vi "Module_IOWrite.vi"(7 "IOWrite_Cmd":T3, 8 "error in (no error)":errorcluster caption="エラー入力", 9 "IOName-LineName":cluster{"IOName":string, "DAQmxChannel":tag}[](array[cluster])=[{"IOName"="BPS_ON", "DAQmxChannel"="PXI1Slot4/port4/line7"}], 10 "ON/OFF":bool, 11 "IOName":string) -> (0 "error out":errorcluster caption="エラー出力", 2 "Check":bool, 3 "IO_State":T1(array[cluster]))   [LabVIEW 2018]
doc: "Module_IOWrite.vi\nIO信号のON/OFF切替を行う。\n\n◆IOWrite_Cmd=Init\n　IO信号制御用DOの初期化処理を行う。\n　また、入力のIO名とLine名の対応を保持する。\n　・Input：IOName-LineName\n\n◆IOWrite_Cmd=Set\n　入力のIONameの信号のON/OFFを切替。\n　・Input：IOName\n　　　　　 ON/OFF\n\n◆IOWrite_Cmd=ALL_OFF\n　全てのIONameの信号をOFFにする。\n\n◆IOWrite_Cmd=Check\n　現在のIO信号の状態を読み出す\n　・Output：IO_State\n\n◆IOWrite_Cmd=Close\n　IO信号信号制御用DOのクローズ処理を行う。"
uses:
  Ctl_IOWriteCommand.ctl
  <vilib>/DAQmx/read.llb/DAQmx Read (Digital 1D Bool NChan 1Samp 1Line).vi
  <vilib>/DAQmx/write.llb/DAQmx Write (Digital 1D Bool NChan 1Samp 1Line).vi
  <vilib>/DAQmx/create/channels.llb/DAQmx Create Channel (DO-Digital Output).vi
  <vilib>/DAQmx/miscellaneous.llb/DAQmx Fill In Error Info.vi
panel:
  in  "IOState":T2={"IOName"="AUTO", "DAQmxChannel"="PXI1Slot4/port0/line0", "ON/OFF"=FALSE}
  # "Output"
  # "Local"
  # "Input"
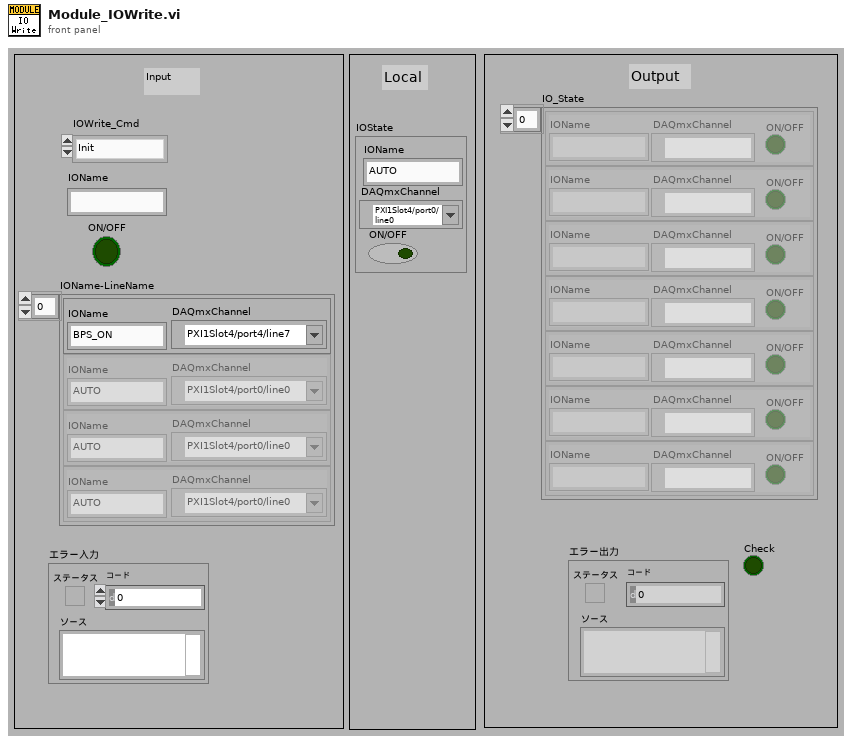
[diagram p1: front panel]
types:
  T1 = cluster{"IOName":string, "DAQmxChannel":tag, "ON/OFF":bool}[]
  T2 = cluster{"IOName":string, "DAQmxChannel":tag, "ON/OFF":bool}
  T3 = typedef "Ctl_IOWriteCommand.ctl" = enum16{"Init", "Set", "ALL_OFF", "Check", "Close"}
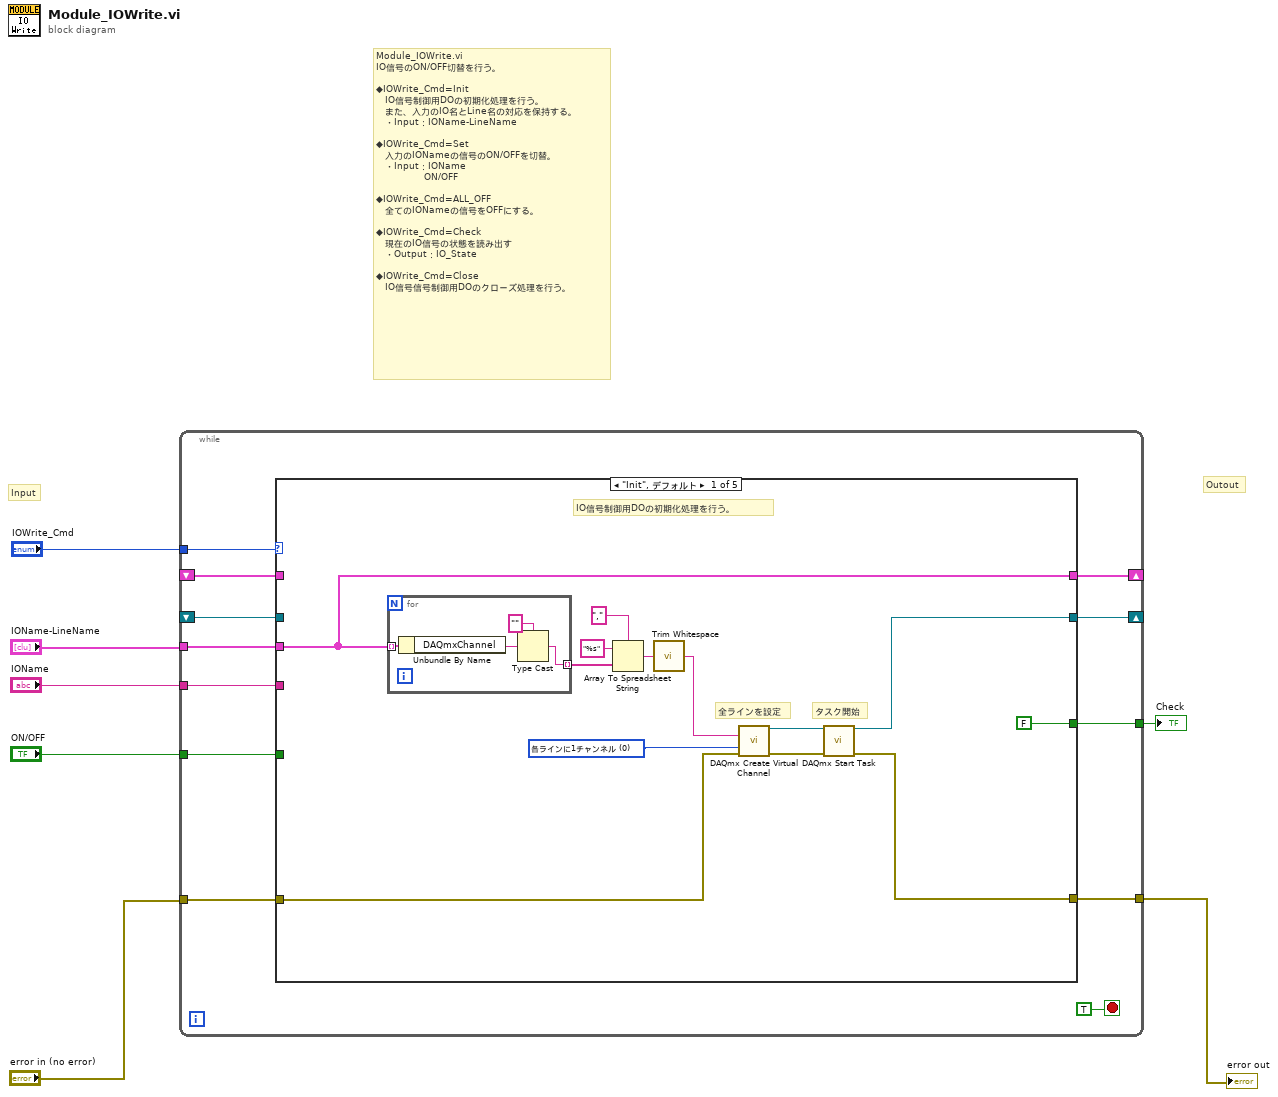
[diagram p0: block diagram]
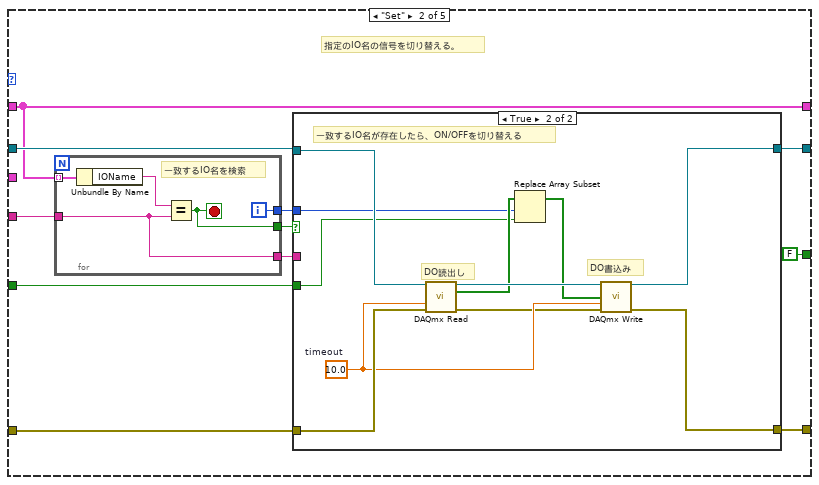
[diagram p2: hidden frame]
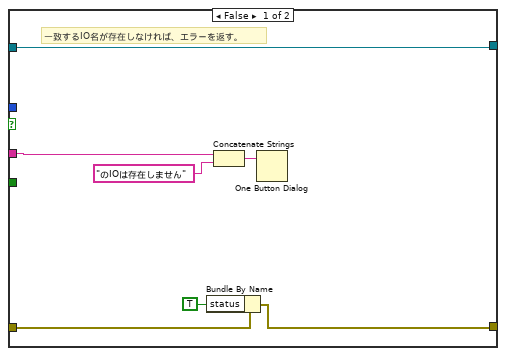
[diagram p3: hidden frame]
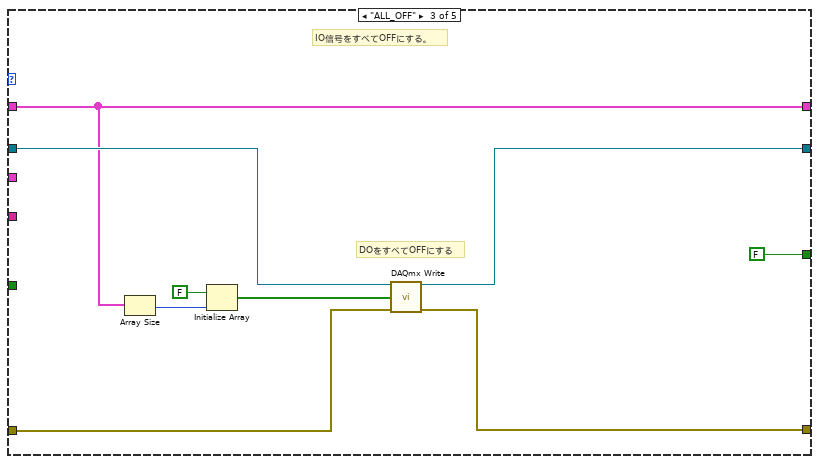
[diagram p4: hidden frame]
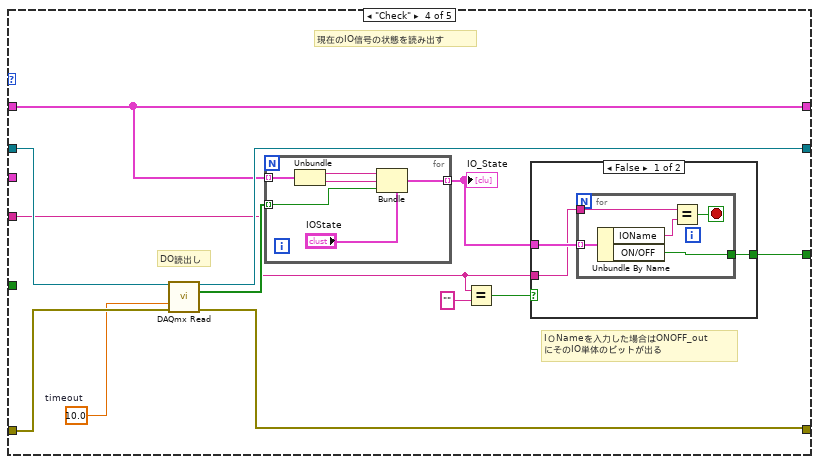
[diagram p5: hidden frame]
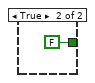
[diagram p6: hidden frame]
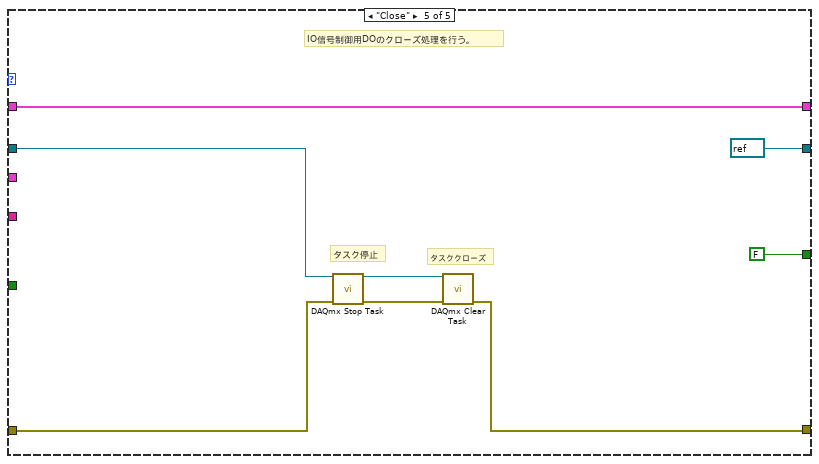
[diagram p7: hidden frame]
diagram:
  # "Module_IOWrite.vi\nIO信号のON/OFF切替を行う。\n\n◆IOWrite_Cmd=Init\n　IO信号制御用DOの初期化処理を行う。\n　また、入力のIO名とLine名の対応を保持する。\n　・Input：IOName-LineName\n\n◆IOWrite_Cmd=Set\n　入力のIONameの信号のON/OFFを切替。\n　・Input：IOName\n　　　　　 ON/OFF\n\n◆IOWrite_Cmd=ALL_OFF\n　全てのIONameの信号をOFFにする。\n\n◆IOWrite_Cmd=Check\n　現在のIO信号の状態を読み出す\n　・Output：IO_State\n\n◆IOWrite_Cmd=Close\n　IO信号信号制御用DOのクローズ処理を行う。"
  # "Outout"
  # "Input"
  n1 = while {
    tunnel: "error in (no error)" -> [w19]
    tunnel: "IOWrite_Cmd" -> [w18]
    shift-right: [w16] -> _
    shift-left: _ -> [w15]
    tunnel: [w8] -> w1
    tunnel: "ON/OFF" -> [w14]
    tunnel: "IOName-LineName" -> [w13]
    tunnel: "IOName" -> [w12]
    shift-right: [w11] -> _
    shift-left: _ -> [w10]
    tunnel: [w9] -> w2
    stop <- TRUE stop-if-true
    n2 = case shown="\"Init\", デフォルト" w18 {
      tunnel: w19 -> [w29 w46 w78 w91 w111]
      tunnel: [w28 w47 w79 w88 refnum<k21> refnum ("task out")] -> w16
      tunnel: w15 -> [_ w45 w77 w90 w112]
      tunnel: [w23 w41 w74 w86 w108] -> w8
      tunnel: w14 -> [_ w44 _ _ _]
      tunnel: w13 -> [w24 _ _ _ _]
      tunnel: w12 -> [_ w43 _ w82 _]
      tunnel: [w24 w38 w72 w85 w109] -> w11
      tunnel: w10 -> [_ w38 w72 w85 w109]
      tunnel: [FALSE ("ON/OFF") FALSE ("ON/OFF") FALSE ("ON/OFF") w83 FALSE ("ON/OFF")] -> w9
      frame "Init", Default {
        w32 = 0 items=["各ラインに1チャンネル", "全てのラインに1チャンネル"] ("line grouping")
        # "全ラインを設定"
        # "IO信号制御用DOの初期化処理を行う。"
        # "タスク開始"
        n3 = for {
          tunnel: w24 -> [w36] mode=indexing
          tunnel: [w33] -> w25 mode=indexing
          n4 = Unbundle By Name(w36) -> ("DAQmxChannel"=w35:tag)
          n5 = Type Cast(type="" ("タイプ"), x=w35) -> (*(type *) &x=w33:string)
        }
        n6 = Array To Spreadsheet String(delimiter (Tab)="," ("デリミタ（タブ）"), array=w25, 3:"%s" ("形式文字列")) -> (spreadsheet string=w22:string)
        n7 = call <vilib>:"Trim Whitespace.vi"("string"=w22) -> ("trimmed string"=w21:string)  [unwired: 1 in]
        n8 = call-poly <vilib>:"DAQmx Create Virtual Channel.vi"("lines"=w21, "line grouping"=w32, "error in"=w29) -> ("task out"=w30:refnum<k21>, "error out"=w31:errorcluster)  [unwired: 11 in]
        n9 = call <vilib>:"DAQmx Start Task.vi"("task/channels in"=w30, "error in"=w31) -> ("task out"=w28:refnum<k21>, "error out"=w23:errorcluster)  [unwired: 12 in]
      }
      frame "Set" {
        # "指定のIO名の信号を切り替える。"
        n10 = for {
          tunnel: w38 -> [w67] mode=indexing
          tunnel: w43 -> [w68]
          tunnel: [w70] -> w42
          tunnel: [w69] -> w40
          tunnel: [w68] -> w39
          i -> [w70]
          stop <- w69 stop-if-true
          # "一致するIO名を検索"
          n11 = Unbundle By Name(w67) -> ("IOName"=w66:string)
          n12 = Equal?(x=w66, y=w68) -> (x = y?=w69:bool)
        }
        n13 = case shown="TRUE" w40 {
          tunnel: [w54 w65] -> w47
          tunnel: w46 -> [w53 w64]
          tunnel: w45 -> [w54 w63]
          tunnel: w44 -> [_ w58]
          tunnel: w42 -> [_ w56]
          tunnel: [w52 w55] -> w41
          tunnel: w39 -> [w50 _]
          frame False {
            # "一致するIO名が存在しなければ、エラーを返す。"
            n14 = Bundle By Name(cluster=w53, "status"=TRUE) -> (w52:errorcluster)
            n15 = Concatenate Strings(w50, "のIOは存在しません" ("文字列")) -> (w48:string)
            n16 = One Button Dialog(message=w48) -> ()  [unwired: 1 in, 1 out]
          }
          frame True {
            w62 = 10.0  # timeout
            # "一致するIO名が存在したら、ON/OFFを切り替える"
            # "DO読出し"
            # "DO書込み"
            n17 = call-poly <vilib>:"DAQmx Read.vi"("task/channels in"=w63, "timeout"=w62, "error in"=w64) -> ("task out"=w60:refnum<k21>, "data"=w59:bool[], "error out"=w61:errorcluster)  [unwired: 10 in]
            n18 = Replace Array Subset(array=w59, new element=w58, index=w56) -> (w57:bool[])
            n19 = call-poly <vilib>:"DAQmx Write.vi"("task/channels in"=w60, "data"=w57, "timeout"=w62, "error in"=w61) -> ("task out"=w65:refnum<k21>, "error out"=w55:errorcluster)  [unwired: 9 in, 1 out]
          }
        }
      }
      frame "ALL_OFF" {
        # "IO信号をすべてOFFにする。"
        # "DOをすべてOFFにする"
        n20 = Array Size(array=w72) -> (size(s)=w73:i32)
        n21 = Initialize Array(FALSE, w73) -> (w75:bool[])
        n22 = call-poly <vilib>:"DAQmx Write.vi"("task/channels in"=w77, "data"=w75, "error in"=w78) -> ("task out"=w79:refnum<k21>, "error out"=w74:errorcluster)  [unwired: 10 in, 1 out]
      }
      frame "Check" {
        w89 = 10.0  # timeout
        # "IＯNameを入力した場合はONOFF_out\nにそのIO単体のビットが出る"
        # "DO読出し"
        # "現在のIO信号の状態を読み出す"
        n23 = call-poly <vilib>:"DAQmx Read.vi"("task/channels in"=w90, "timeout"=w89, "error in"=w91) -> ("task out"=w88:refnum<k21>, "data"=w87:bool[], "error out"=w86:errorcluster)  [unwired: 10 in]
        n24 = for {
          tunnel: w85 -> [w104] mode=indexing
          tunnel: w87 -> [w106] mode=indexing
          tunnel: [w101] -> w84 mode=indexing
          n25 = Unbundle(w104) -> ("IOName"=w103:string, "DAQmxChannel"=w102:tag)
          n26 = Bundle(cluster="IOState", "IOName"=w103, "DAQmxChannel"=w102, "ON/OFF"=w106) -> (w101:T2)
        }
        "IO_State" <- w84
        n27 = Equal?(x=w82, y="") -> (x = y?=w80:bool)
        n28 = case shown="FALSE" w80 {
          tunnel: w84 -> [w94 _]
          tunnel: w82 -> [w93 _]
          tunnel: [w92 FALSE ("ON/OFF")] -> w83
          frame False {
            n29 = for {
              tunnel: [w99] -> w92
              tunnel: w94 -> [w96] mode=indexing
              tunnel: w93 -> [w95]
              stop <- w97 stop-if-true
              n30 = Unbundle By Name(w96) -> ("IOName"=w98:string, "ON/OFF"=w99:bool)
              n31 = Equal?(x=w95, y=w98) -> (x = y?=w97:bool)
            }
          }
          frame True {
          }
        }
      }
      frame "Close" {
        # "タスククローズ"
        # "タスク停止"
        # "IO信号制御用DOのクローズ処理を行う。"
        n32 = call <vilib>:"DAQmx Stop Task.vi"("task/channels in"=w112, "error in"=w111) -> ("task out"=w114:refnum<k21>, "error out"=w113:errorcluster)  [unwired: 12 in]
        n33 = call <vilib>:"DAQmx Clear Task.vi"("task in"=w114, "error in"=w113) -> ("error out"=w108:errorcluster)  [unwired: 13 in]
      }
    }
  }
  "error out" <- w1
  "Check" <- w2
